vi "GenerateData.vi"(8 "error in (no error)":errorcluster, 11 "Camera_Prime95B in":refnum<class "Camera_Prime95B.lvclass">) -> (0 "error out":errorcluster, 2 "DataExchange":T1, 3 "Camera_Prime95B out":refnum<class "Camera_Prime95B.lvclass">)   [LabVIEW 2020]
uses:
  Camera_Prime95B.lvclass
  Hardware Abstraction Layer/Component/Device/Device/DataExchange.ctl
  Interface/DataListener/DataListener.lvclass
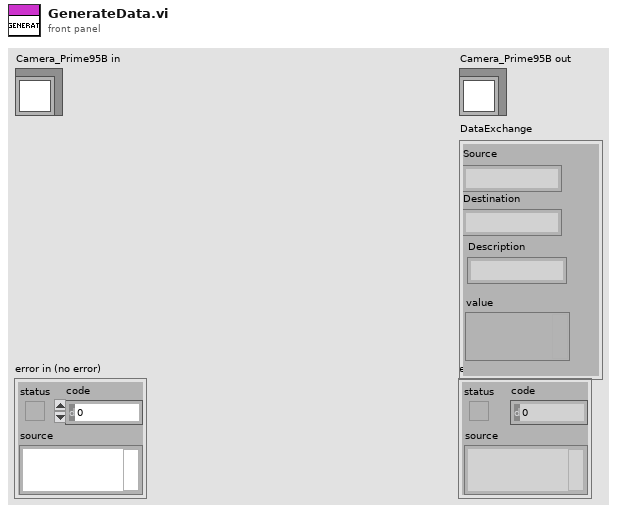
[diagram p1: front panel]
types:
  T1 = typedef "DataListener.lvclass/DataExchange.ctl" = cluster{"Source":string, "Destination":string, "Description":string, "value":variant}
  T2 = typedef "IMAQ Image.ctl" = refnum<image>
  T3 = typedef "Image Type" = u32
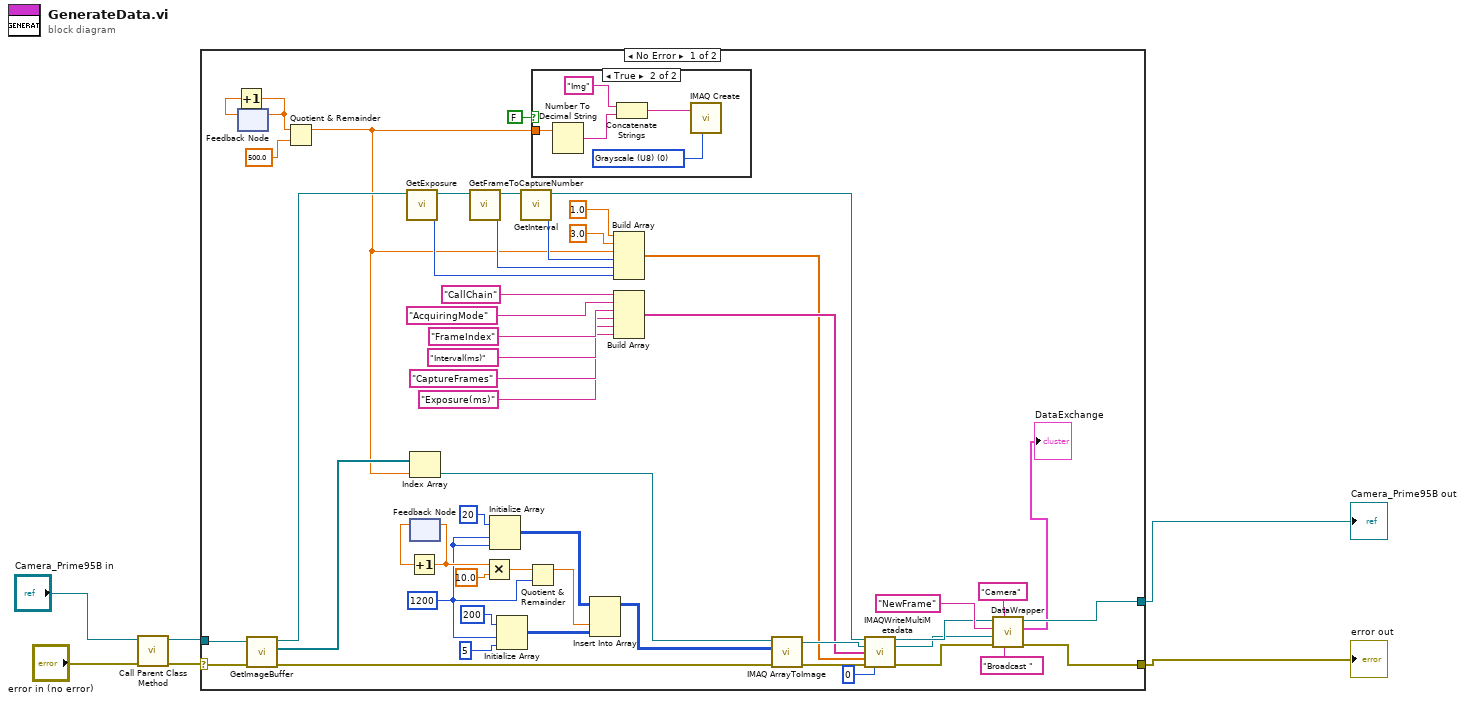
[diagram p0: block diagram]
diagram:
  n1 = call-parent "Call Parent Class Method"("error in (no error)"="error in (no error)", "GRMActor in"="Camera_Prime95B in") -> ("error out"=w4:errorcluster, "GRMActor out"=w3:refnum<class "Camera_Prime95B.lvclass">)  [unwired: 7 in, 1 out]
  n2 = case shown="No Error" w4 {
    selector: w4 -> [w39 w64]
    tunnel: [w38 w64] -> w1
    tunnel: [w47 w63] -> w2
    tunnel: w3 -> [w15 w63]
    frame No Error {
      w41 = 1200 ("dimension size")
      n3 = feedback #1() -> (w48:dbl)  [unwired: 1 in]
      n4 = Increment(x=w48) -> (x+1=w10:dbl)
      n5 = feedback-in #1(w10) -> ()
      n6 = call-dynamic "GetImageBuffer.vi"("error in (no error)"=w39, "Camera in"=w15) -> ("error out"=w16:errorcluster, "ImageBuffer"=w12:T2[], "Camera out"=w14:refnum<class "Camera_Prime95B.lvclass">)  [unwired: 6 in, 1 out]
      n7 = Quotient & Remainder(x=w10, y=500.0) -> (x-y*floor(x/y)=w8:dbl)  [unwired: 1 out]
      n8 = call-dynamic "GetExposure.vi"("Camera in"=w14) -> ("Setting.Exposure"=w18:i32, "Camera out"=w37:refnum<class "Camera_Prime95B.lvclass">)  [unwired: 8 in, 1 out]
      n9 = Index Array(array=w12, index=w8) -> (element=w11:T2)
      n10 = feedback #2() -> (w46:dbl)  [unwired: 1 in]
      n11 = Increment(x=w46) -> (x+1=w44:dbl)
      n12 = feedback-in #2(w44) -> ()
      n13 = call-dynamic "GetFrameToCaptureNumber.vi"("Camera in"=w37) -> ("Setting.FramesToCapture"=w22:i32, "Camera out"=w36:refnum<class "Camera_Prime95B.lvclass">)  [unwired: 8 in, 1 out]
      n14 = Multiply(x=w44, y=10.0) -> (x*y=w43:dbl)
      n15 = Initialize Array(u64 20 ("element"), w41, w41) -> (w56:u64[][])
      n16 = Initialize Array(u64 200 ("element"), w41, 5 ("dimension size")) -> (w53:u64[][])
      n17 = call-dynamic "GetInterval.vi"("Camera in"=w36) -> ("Setting.Interval"=w19:i32, "Camera out"=w26:refnum<class "Camera_Prime95B.lvclass">)  [unwired: 8 in, 1 out]
      n18 = Quotient & Remainder(x=w43, y=w41) -> (x-y*floor(x/y)=w45:dbl)  [unwired: 1 out]
      n19 = case shown="True" FALSE {
        tunnel: w8 -> [_ w58]
        frame False {
        }
        frame True {
          w62 = T3 0 items=["Grayscale (U8)", "Grayscale (I16)", "Grayscale (SGL)", "Complex (CSG)", "RGB (U32)", "HSL (U32)", "RGB (U64)", "Grayscale (U16)"] ("Image Type")
          n20 = Number To Decimal String(number=w58) -> (decimal integer string=w59:string)  [unwired: 1 in]
          n21 = Concatenate Strings("Img" ("Image Name"), w59) -> (w60:string)
          n22 = call "IMAQ Create"("Image Name"=w60, "Image Type"=w62) -> ()  [unwired: 3 in, 2 out]
        }
      }
      n23 = Insert Into Array(array=w56, index (col)=w45, new element=w53) -> (w55:u64[][])  [unwired: 1 in]
      n24 = Build Array(1.0 ("y"), 3.0 ("y"), w8, w19, w22, w18) -> (w20:dbl[])
      n25 = Build Array("CallChain" ("Key"), "AcquiringMode" ("Key"), "FrameIndex" ("Key"), "Interval(ms)" ("Key"), "CaptureFrames" ("Key"), "Exposure(ms)" ("Key")) -> (w21:string[])
      n26 = call "IMAQ ArrayToImage"("error in (no error)"=w16, "Image Pixels (U8)"=w55, "Image"=w11) -> ("error out"=w49:errorcluster, "Image Out"=w24:T2)  [unwired: 7 in]
      n27 = call-dynamic "IMAQWriteMultiMetadata.vi"("GRMActor in"=w26, "Image In"=w24, "Keys"=w21, "Values"=w20, "error in (no error)"=w49, "precision (6)"=i16 0) -> ("GRMActor out"=w25:refnum<class "Camera_Prime95B.lvclass">, "Image Out"=w23:T2, "error out"=w27:errorcluster)  [unwired: 7 in]
      n28 = call-dynamic "DataWrapper.vi"("Destination"="Broadcast " ("Type"), "Source"="Camera", "error in (no error)"=w27, "value"=w23, "Description"="NewFrame" ("Target"), "GRMActor in"=w25) -> ("error out"=w38:errorcluster, "DataExchange"=→"DataExchange":T1, "GRMActor out"=w47:refnum<class "Camera_Prime95B.lvclass">)  [unwired: 3 in]
    }
    frame Error {
    }
  }
  "error out" <- w1
  "Camera_Prime95B out" <- w2
